vi "calibrationElectrometer_putSample_Intensity.vi"(8 "error in (no error)":errorcluster, 11 "Intensity_Ctl":T1) -> (0 "error out":errorcluster, 2 "function return":i32, 3 "Intensity_Ctl out":T1)   [LabVIEW 2016, in "SALLV_calibrationElectrometer.lvlib"]
doc: "int calibrationElectrometer_shm_putSample_IntensityLV(calibrationElectrometer_IntensityLV *Intensity_Ctl );"
uses:
  SALLV_calibrationElectrometer.lvlib
  DataTypes/Intensity.ctl
  SALLV_calibrationElectrometer.so
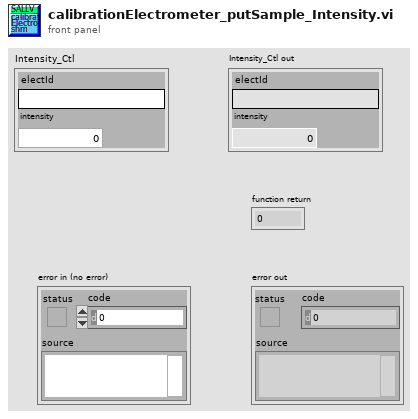
[diagram p1: front panel]
types:
  T1 = typedef "SALLV_calibrationElectrometer.lvlib/Intensity.ctl" = cluster{"electId":string, "intensity":dbl}
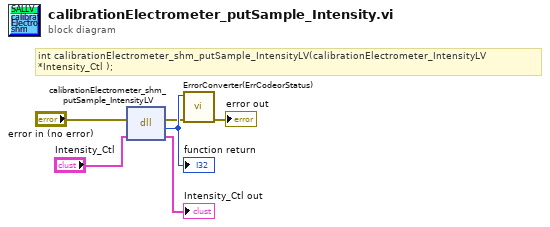
[diagram p0: block diagram]
diagram:
  # "int calibrationElectrometer_shm_putSample_IntensityLV(calibrationElectrometer_IntensityLV *Intensity_Ctl );"
  n1 = dll-call lib="home/harini/tcs/ts_SALLV_calibrationElectrometer/SALLV_calibrationElectrometer.*" fn="calibrationElectrometer_shm_putSample_IntensityLV"(error in="error in (no error)", "Intensity_Ctl"="Intensity_Ctl") -> (error out=w2:errorcluster, w6:i32, "Intensity_Ctl"=→"Intensity_Ctl out":T1)  [unwired: 2 in, 1 out]
  "function return" <- w6
  n2 = call "ErrorConverter(ErrCodeorStatus).vi"("error in (no error)"=w2, "error code"=w6) -> ("error out"=→"error out":errorcluster)  [unwired: 9 in]
